vi "SPI_Open.vi"(5 "Device":i32, 7 "Bus":i32=1, 8 "error in":errorcluster) -> (0 "error out":errorcluster)   [LabVIEW 2014]
doc: "Opens the specified device"
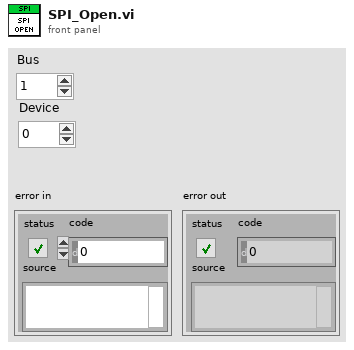
[diagram p1: front panel]
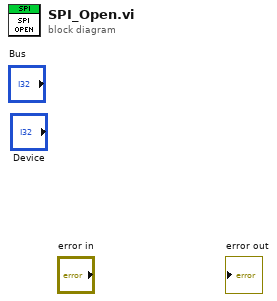
[diagram p0: block diagram]
diagram:
